vi "py File Name.vi"(0 "Path":path, 11 "error in (no error)":errorcluster) -> (4 "String":string, 15 "error out":errorcluster)   [LabVIEW 2016, in "Py Doc.lvclass"]
uses:
  Py Doc.lvclass
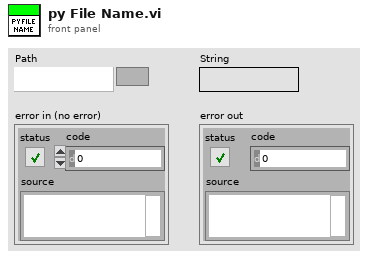
[diagram p1: front panel]
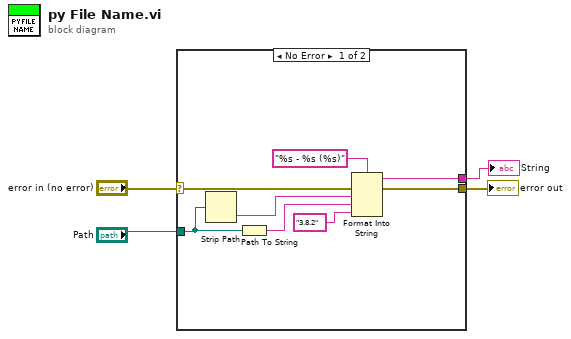
[diagram p0: block diagram]
diagram:
  n1 = case shown="No Error" "error in (no error)" {
    selector: "error in (no error)" -> [w6 w13]
    tunnel: "Path" -> [w12 _]
    tunnel: [w10 _] -> w3
    tunnel: [w5 w13] -> w1
    frame No Error {
      n2 = Strip Path(path=w12) -> (name=w7:string)  [unwired: 1 out]
      n3 = Path To String(path=w12) -> (string=w11:string)
      n4 = Format Into String(format string="%s - %s (%s)", error in=w6, w7, w11, "3.8.2" ("input 3")) -> (resulting string=w10:string, error out=w5:errorcluster)  [unwired: 1 in]
    }
    frame Error {
    }
  }
  "String" <- w3
  "error out" <- w1
